vi "Eth Status Manager Init.vi"(8 "error in (no error)":errorcluster, 11 "Data Buffer Length":i32=1000) -> (0 "error out":errorcluster, 3 "Status Reference":T1)   [LabVIEW 2021, in "Eth Status.lvlib"]
uses:
  Eth Status.lvlib
  Ctl/Status.ctl
  MB_TCP2/MB_TCP_State.ctl
  MB_TCP2/MB_TCP.lvclass
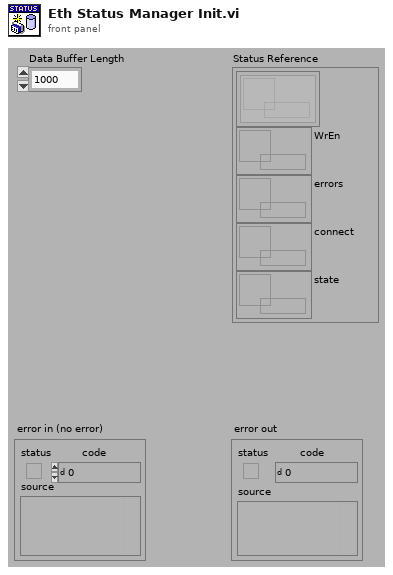
[diagram p1: front panel]
types:
  T1 = typedef "Eth Status.lvlib/Status.ctl" = cluster{"Set_states":refnum<queue>[], "WrEn":refnum<data-value>, "errors":refnum<data-value>, "connect":refnum<data-value>, "state":refnum<data-value>}
  T2 = typedef "MB_TCP.lvclass/MB_TCP_State.ctl" = enum8{"initialization", "redefine", "standby", "connect", "wait to reconnect", "wait to reset timeout", "configure", "requests", "close connection", "stop"}
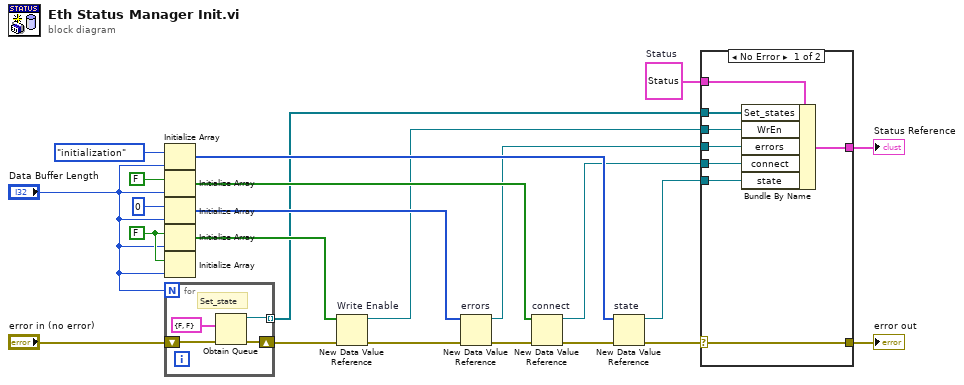
[diagram p0: block diagram]
diagram:
  w16 = FALSE
  w23 = T1 {"Set_states"=[], "WrEn"=refnum, "errors"=refnum, "connect"=refnum, "state"=refnum}  # Status
  n1 = Initialize Array(MB_TCP_State."initialization" ("MB_TCP_State"), "Data Buffer Length") -> (w12:T2[])
  n2 = Initialize Array(FALSE, "Data Buffer Length") -> (w15:bool[])
  n3 = Initialize Array(0, "Data Buffer Length") -> (w22:i32[])
  n4 = Initialize Array(w16, "Data Buffer Length") -> (w17:bool[])
  n5 = Initialize Array(w16, "Data Buffer Length") -> ()  [unwired: 1 out]
  n6 = for {
    N: "Data Buffer Length" -> [_]
    shift-right: [w25] -> w4
    shift-left: "error in (no error)" -> [w26]
    tunnel: [w24] -> w1 mode=indexing
    # "Set_state"
    n7 = Obtain Queue(element data type=cluster{"Start":bool, "Stop":bool} {"Start"=FALSE, "Stop"=FALSE} ("Set_state"), error in (no error)=w26) -> (queue out=w24:refnum<queue>, error out=w25:errorcluster)  [unwired: 3 in, 1 out]
  }
  n8 = New Data Value Reference "Write Enable"(data value=w17, error in=w4) -> (data value reference=w10:refnum<data-value>, error out=w5:errorcluster)
  n9 = New Data Value Reference "errors"(data value=w22, error in=w5) -> (data value reference=w9:refnum<data-value>, error out=w11:errorcluster)
  n10 = New Data Value Reference "connect"(data value=w15, error in=w11) -> (data value reference=w8:refnum<data-value>, error out=w7:errorcluster)
  n11 = New Data Value Reference "state"(data value=w12, error in=w7) -> (data value reference=w6:refnum<data-value>, error out=w20:errorcluster)
  n12 = case shown="No Error" w20 {
    selector: w20 -> [w34 w36]
    tunnel: w23 -> [w29 w37]
    tunnel: [w35 w37] -> w21
    tunnel: [w34 w36] -> w19
    tunnel: w10 -> [w33 _]
    tunnel: w9 -> [w32 _]
    tunnel: w8 -> [w31 _]
    tunnel: w6 -> [w30 _]
    tunnel: w1 -> [w28 _]
    frame No Error {
      n13 = Bundle By Name(cluster=w29, "Set_states"=w28, "WrEn"=w33, "errors"=w32, "connect"=w31, "state"=w30) -> (w35:T1)
    }
    frame Error {
    }
  }
  "error out" <- w19
  "Status Reference" <- w21
